vi "Call Check Previous Values.vi"(8 "error in":errorcluster, 10 "values":dbl[](array[numeric]), 11 "Tx Scheduled Labels Execution Unit in":refnum<class "Tx Scheduled Labels Execution Unit.lvclass">) -> (0 "error out":errorcluster, 1 "modified indices":i32[](array[numeric]), 2 "values out":dbl[](array[numeric]), 3 "Tx Scheduled Labels Execution Unit out":refnum<class "Tx Scheduled Labels Execution Unit.lvclass">, 4 "values modified?":bool)   [LabVIEW 2020, in "Ballard ARINC 429 Engine.lvlib" / "Implementation.lvlib" / "Tx Scheduled Labels Execution Unit.lvclass"]
uses:
  Tx Scheduled Labels Execution Unit.lvclass
  Tx Scheduled Labels Execution Unit.lvclass/Tx Scheduled Labels Execution Unit.ctl
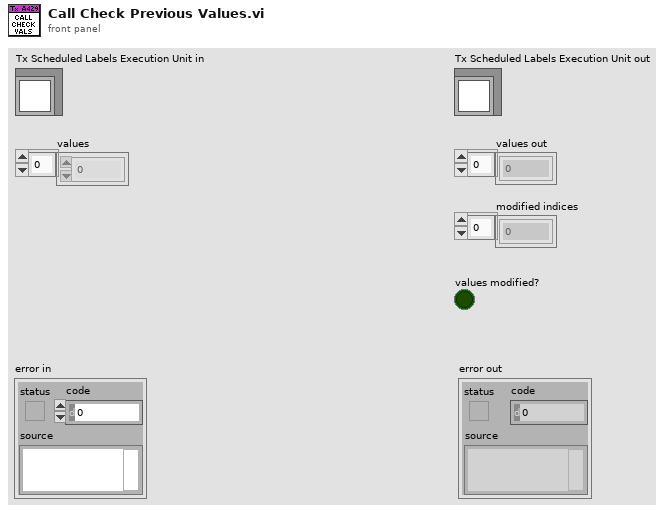
[diagram p1: front panel]
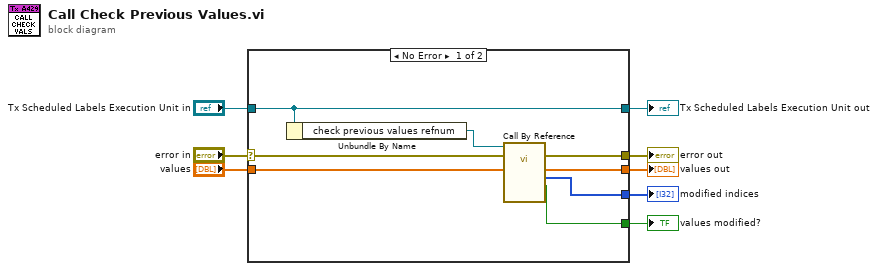
[diagram p0: block diagram]
diagram:
  n1 = case shown="No Error" "error in" {
    selector: "error in" -> [w10 w19]
    tunnel: [w9 w19] -> w7
    tunnel: [w16 w18] -> w5
    tunnel: "Tx Scheduled Labels Execution Unit in" -> [w16 w18]
    tunnel: "values" -> [w14 w17]
    tunnel: [w13 w17] -> w3
    tunnel: [w12 _] -> w2
    tunnel: [w11 _] -> w1
    frame No Error {
      n2 = Unbundle By Name(w16) -> ("check previous values refnum"=w15:refnum<vi>)
      n3 = call-by-ref "?"(reference=w15, error in=w10, "values"=w14) -> (error out=w9:errorcluster, "values modified?"=w11:bool, "modified indices"=w12:i32[], "values out"=w13:dbl[])  [unwired: 8 in, 1 out]
    }
    frame Error {
    }
  }
  "error out" <- w7
  "Tx Scheduled Labels Execution Unit out" <- w5
  "values out" <- w3
  "modified indices" <- w2
  "values modified?" <- w1
